vi "Verify Hello World.vi"(11 "Test Case In":refnum<class "Simple Tests.lvclass">) -> (0 "error out":errorcluster, 3 "Test Case Out":refnum<class "Simple Tests.lvclass">)   [LabVIEW 2020, in "Simple Tests.lvclass"]
uses:
  Simple Tests.lvclass
  C:/Program Files/National Instruments/LabVIEW 2026/vi.lib/Astemes/LUnit/Test Case.lvclass
  <vilib>/SAS/Approval Tests/Approval Tests/Options/Options.lvclass/Options.ctl
  <vilib>/SAS/Approval Tests/Approval Tests/Naming Data/Naming Data.lvclass/Naming Data.ctl
  <vilib>/Astemes/LUnit/Test Case.lvclass/Test Case.ctl
  <vilib>/SAS/Approval Tests/Approval Tests/Options/Options.lvclass
  <vilib>/SAS/Approval Tests/Approval Tests/Scrubber/Scrubber.lvclass
  <vilib>/SAS/Approval Tests/Approval Tests/Namer/Namer.lvclass
  <vilib>/SAS/Approval Tests/Approval Tests/Naming Data/Naming Data.lvclass
  <vilib>/SAS/Approval Tests/Approval Tests/Reporter/Reporter.lvclass
  <vilib>/SAS/Approval Tests/Approval Tests/Text Comparator/Text Comparator.lvclass
  e8482912-3f63-4122-8bd4-83730cc6f185.vi
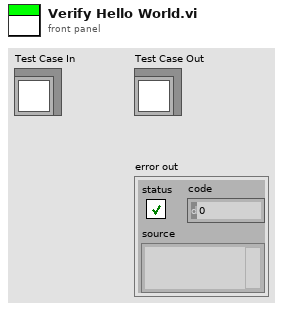
[diagram p1: front panel]
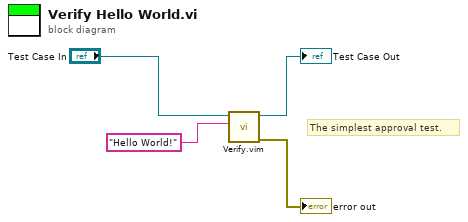
[diagram p0: block diagram]
diagram:
  # "The simplest approval test."
  n1 = call "Verify.vim"("Test Data"="Hello World!", "LUnit Test Case In"="Test Case In") -> ("error out"=→"error out":errorcluster, "LUnit Test Case Out"=→"Test Case Out":refnum<class "Simple Tests.lvclass">)  [unwired: 8 in]
